vi "Bounds - thread count.vi"(8 "error in (no error)":errorcluster, 11 "lvzstd in":refnum<class "lvzstd.lvclass">) -> (0 "error out":errorcluster, 1 "max_count":i32, 2 "min_count":i32, 3 "lvzstd out":refnum<class "lvzstd.lvclass">)   [LabVIEW 2020, in "lvzstd.lvlib" / "lvzstd.lvclass"]
uses:
  lvzstd.lvclass
  lvzstd.lvclass/lvzstd.ctl
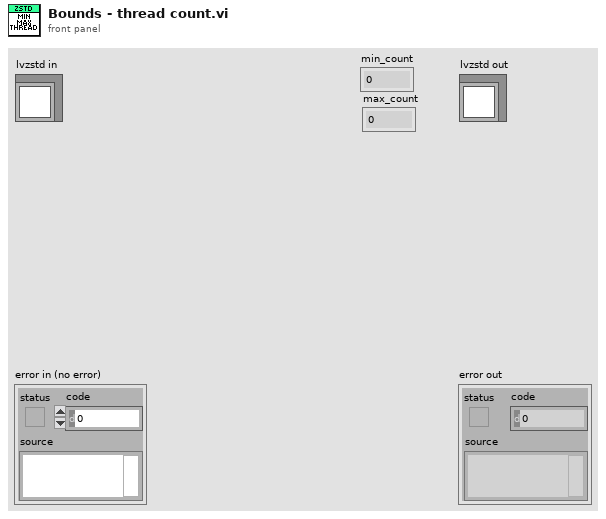
[diagram p1: front panel]
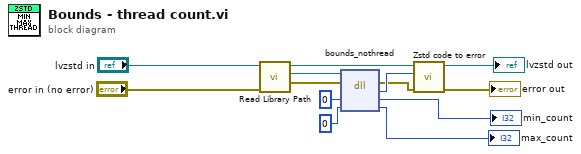
[diagram p0: block diagram]
diagram:
  n1 = call "Read Library Path.vi"("error in (no error)"="error in (no error)", "lvzstd in"="lvzstd in") -> ("error out"=w10:errorcluster, "Library Path"=w11:path, "lvzstd out"=w5:refnum<class "lvzstd.lvclass">)  [unwired: 7 in]
  n2 = dll-call lib="?" fn="bounds_nothread"(path in=w11, error in=w10, "min_count"=0, "max_count"=0 ("max_compressed_size")) -> (error out=w2:errorcluster, "return type"=w3:i32, "min_count"=→"min_count":i32, "max_count"=→"max_count":i32)  [unwired: 1 in, 1 out]
  n3 = call "Zstd code to error.vi"("error in"=w2, "Error code"=w3, "lvzstd in"=w5) -> ("error in (no error)"=→"error out":errorcluster, "lvzstd out"=→"lvzstd out":refnum<class "lvzstd.lvclass">)  [unwired: 7 in]
